vi "DAQ.Auto Configure.vi"(8 "error in (no error)":errorcluster, 11 "Instrument.DAQ":refnum<class "Instrument.DAQ.lvclass">) -> (0 "error out":errorcluster, 3 "Instrument.DAQ out":refnum<class "Instrument.DAQ.lvclass">)   [LabVIEW 2019, in "Instrument.Lockin.lvlib" / "Instrument.DAQ.lvclass"]
uses:
  Instrument.DAQ.lvclass
  DAQmx/typedefs/DAQmx.Commands--enum.ctl
  Instrument.DAQ.lvclass/Instrument.DAQ.ctl
  DAQmx/DAQmx.lvclass
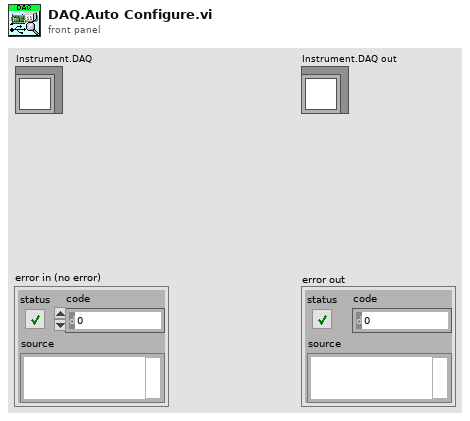
[diagram p1: front panel]
types:
  T1 = typedef "DAQmx.lvclass/DAQmx.Commands--enum.ctl" = enum16{"idle", "start", "stop", "calibrate", "auto", "exit"}
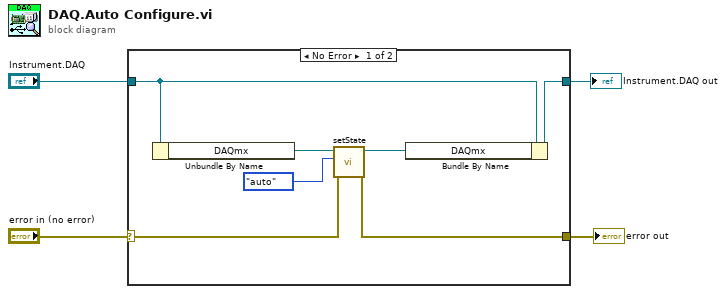
[diagram p0: block diagram]
diagram:
  n1 = case shown="No Error" "error in (no error)" {
    selector: "error in (no error)" -> [w8 w12]
    tunnel: [w7 w12] -> w4
    tunnel: "Instrument.DAQ" -> [w11 w13]
    tunnel: [w6 w13] -> w2
    frame No Error {
      n2 = Unbundle By Name(w11) -> ("DAQmx"=w10:refnum<class "DAQmx.lvclass">)
      n3 = call "setState.vi"("error in (no error)"=w8, "Command"=DAQmx.Commands--enum."auto" ("State"), "DAQmx in"=w10) -> ("error out"=w7:errorcluster, "DAQmx out"=w9:refnum<class "DAQmx.lvclass">)  [unwired: 7 in]
      n4 = Bundle By Name(cluster=w11, "DAQmx"=w9) -> (w6:refnum<class "Instrument.DAQ.lvclass">)
    }
    frame Error {
    }
  }
  "error out" <- w4
  "Instrument.DAQ out" <- w2
